vi "LJT4_stream_read.vi"(8 "error in":errorcluster, 9 "NumReadAddresses":i32, 10 "ScansPerRead":i32, 11 "Handle in":i32) -> (0 "error out":errorcluster, 3 "Handle Out":i32, 4 "status":bool, 5 "data_out":dbl[][](array[numeric]))   [LabVIEW 2019]
panel:
  out "DeviceScanBacklog":i32
  out "LJMScanBacklog":i32
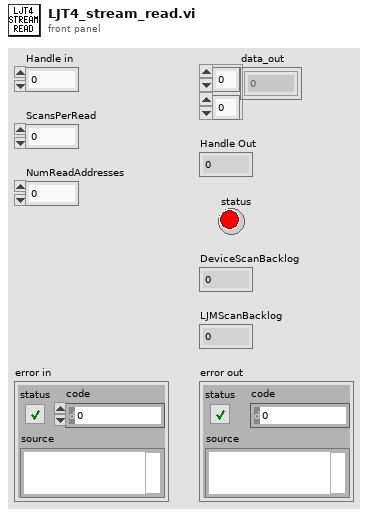
[diagram p1: front panel]
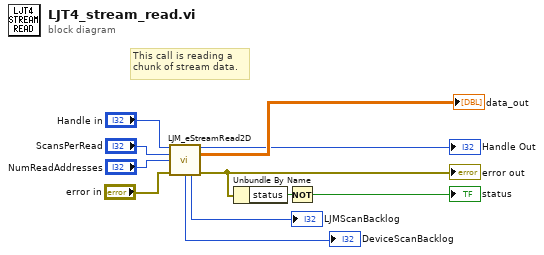
[diagram p0: block diagram]
diagram:
  # "This call is reading a\nchunk of stream data."
  n1 = call "LJM_eStreamRead2D.vi"("Handle In"="Handle in", "ScansPerRead"="ScansPerRead", "NumAddresses"="NumReadAddresses", "error in"="error in") -> ("Handle Out"=→"Handle Out":i32, "aData Out"=→"data_out":dbl[][], "DeviceScanBacklog"=→"DeviceScanBacklog":i32, "LJMScanBacklog"=→"LJMScanBacklog":i32, "error out"=w8:errorcluster)  [unwired: 7 in]
  "error out" <- w8
  n2 = Unbundle By Name(w8) -> ("status"=w2:bool)
  n3 = Not(x=w2) -> (.not. x?=→"status":bool)
